vi "build_array.vi"() -> ()   [LabVIEW 2021]
panel:
  out "Array 3":i32[](array[numeric])
  out "time 3":u32
  out "Array 2":i32[](array[numeric])
  out "time 2":u32
  out "time":u32
  out "Array":i32[](array[numeric])
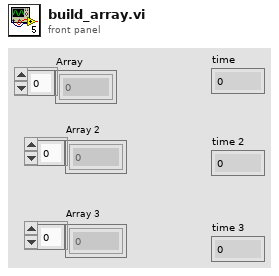
[diagram p1: front panel]
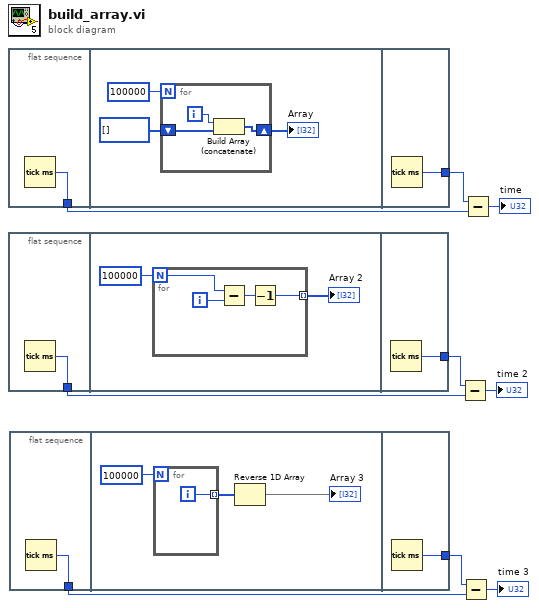
[diagram p0: block diagram]
diagram:
  n1 = flat-sequence {
    tunnel: [w10] -> w8
    tunnel: [w17] -> w9
    frame #0 {
      n2 = Tick Count (ms)() -> (millisecond timer value=w10:u32)
    }
    frame #1 {
      n3 = for {
        N: 100000 -> [_]
        shift-right: [w14] -> w11
        shift-left: i32[] [] -> [w15]
        i -> [w16]
        n4 = Build Array (concatenate)(w16, w15) -> (w14:i32[])
      }
      "Array" <- w11
    }
    frame #2 {
      n5 = Tick Count (ms)() -> (millisecond timer value=w17:u32)
    }
  }
  n6 = flat-sequence {
    tunnel: [w18] -> w5
    tunnel: [w25] -> w4
    frame #0 {
      n7 = Tick Count (ms)() -> (millisecond timer value=w18:u32)
    }
    frame #1 {
      n8 = for {
        N: 100000 -> [w24]
        tunnel: [w21] -> w19 mode=indexing
        i -> [w23]
        n9 = Subtract(x=w24, y=w23) -> (x-y=w22:i32)
        n10 = Decrement(x=w22) -> (x-1=w21:i32)
      }
      "Array 2" <- w19
    }
    frame #2 {
      n11 = Tick Count (ms)() -> (millisecond timer value=w25:u32)
    }
  }
  n12 = flat-sequence {
    tunnel: [w26] -> w2
    tunnel: [w31] -> w3
    frame #0 {
      n13 = Tick Count (ms)() -> (millisecond timer value=w26:u32)
    }
    frame #1 {
      n14 = for {
        N: 100000 -> [_]
        tunnel: [w30] -> w28 mode=indexing
        i -> [w30]
      }
      n15 = Reverse 1D Array(array=w28) -> (reversed array=→"Array 3":i32[])
    }
    frame #2 {
      n16 = Tick Count (ms)() -> (millisecond timer value=w31:u32)
    }
  }
  n17 = Subtract(x=w4, y=w5) -> (x-y=→"time 2":u32)
  n18 = Subtract(x=w3, y=w2) -> (x-y=→"time 3":u32)
  n19 = Subtract(x=w9, y=w8) -> (x-y=→"time":u32)
